vi "TDC_getCurrentAddress.vi"(8 "Error In":errorcluster) -> (0 "Error Out":errorcluster, 3 "Device Number":i32)   [LabVIEW 2011]
uses:
  tdcbase.dll
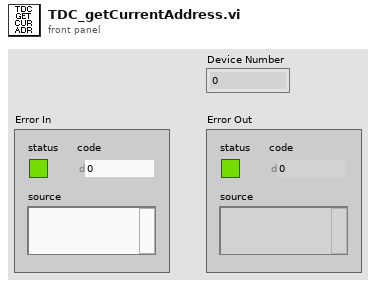
[diagram p1: front panel]
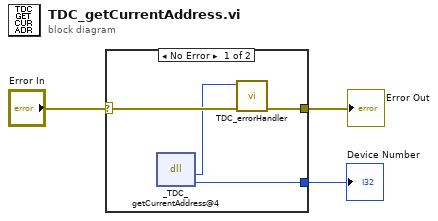
[diagram p0: block diagram]
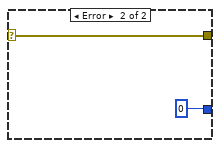
[diagram p2: hidden frame]
diagram:
  n1 = case shown="No Error" "Error In" {
    selector: "Error In" -> [w7 w9]
    tunnel: [w6 w9] -> w2
    tunnel: [w4 0] -> w1
    frame No Error {
      n2 = dll-call lib="X:/tdcbase.dll" fn="_TDC_getCurrentAddress@4"() -> ("return type"=w5:i32, "devNo"=w4:i32)  [unwired: 4 in, 2 out]
      n3 = call "TDC_errorHandler.vi"("Error In"=w7, "TDC Return Code"=w5) -> ("Error Out"=w6:errorcluster)  [unwired: 9 in]
    }
    frame Error {
    }
  }
  "Error Out" <- w2
  "Device Number" <- w1
